vi "5-2 Cluster Experiment.vi"() -> ()   [LabVIEW 2014]
panel:
  out "Small Cluster":cluster{"Boolean 2":bool, "Slide Value":dbl}
  out "Modified Cluster":T1 {"Slide" scale=0.0..10.0}
  in  "Cluster":T1 {"Slide" scale=0.0..10.0}
  out "Boolean":bool
  out "Numeric":dbl
  in  "stop":bool
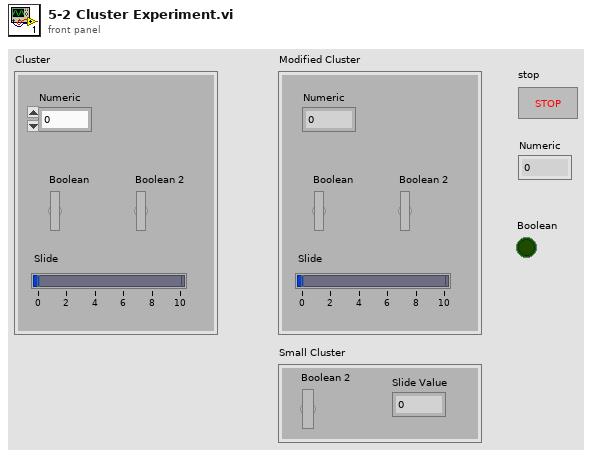
[diagram p1: front panel]
types:
  T1 = cluster{"Numeric":dbl, "Boolean":bool, "Boolean 2":bool, "Slide":dbl}
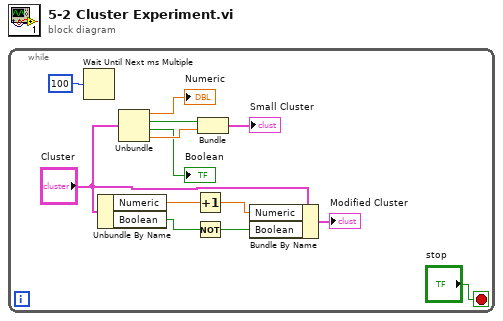
[diagram p0: block diagram]
diagram:
  n1 = while {
    stop <- "stop" stop-if-true
    n2 = Wait Until Next ms Multiple(millisecond multiple=u32 100) -> ()  [unwired: 1 out]
    n3 = Unbundle By Name("Cluster") -> ("Numeric"=w5:dbl, "Boolean"=w2:bool)
    n4 = Unbundle("Cluster") -> ("Numeric"=→"Numeric":dbl, "Boolean"=w11:bool, "Boolean 2"=→"Boolean":bool, "Slide"=w10:dbl)
    n5 = Increment(x=w5) -> (x+1=w4:dbl)
    n6 = Not(x=w2) -> (.not. x?=w1:bool)
    n7 = Bundle("Boolean"=w11, "Slide"=w10) -> (→"Small Cluster":cluster{"Boolean":bool, "Slide":dbl})  [unwired: 1 in]
    n8 = Bundle By Name(cluster="Cluster", "Numeric"=w4, "Boolean"=w1) -> (→"Modified Cluster":T1)
  }
